vi "Single Char Seperator.vi"(8 "error in (no error)":errorcluster, 10 "String":string, 11 "VISA resource name":refnum<visa-resource-name>) -> (0 "error out":errorcluster, 3 "VISA resource name 2":refnum<visa-resource-name>)   [LabVIEW 2013]
panel:
  out "return count":u32
  # "This progarm seperates out strings of commands into single\ncharacters and writes them to the buffer one at a time.  Last I\nchecked, this worked fine.  It is possible that this may not be \nneeded in the future."
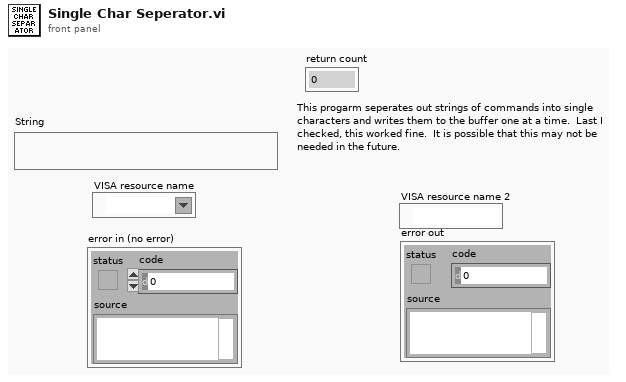
[diagram p1: front panel]
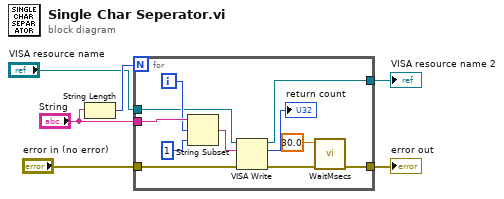
[diagram p0: block diagram]
diagram:
  n1 = String Length(string="String") -> (length=w6:i32)
  n2 = for {
    N: w6 -> [_]
    tunnel: "String" -> [w17]
    tunnel: "VISA resource name" -> [w14]
    tunnel: "error in (no error)" -> [w13]
    tunnel: [w12] -> w2
    tunnel: [w8] -> w1
    i -> [w16]
    n3 = String Subset(string=w17, offset (0)=w16, length (rest)=1 ("length (rest)")) -> (substring=w11:string)
    n4 = VISA Write(VISA resource name=w14, write buffer=w11, error in (no error)=w13) -> (VISA resource name out=w12:refnum<visa-resource-name>, return count=→"return count":u32, error out=w9:errorcluster)
    n5 = call "WaitMsecs.vi"("error in (no error)"=w9, "Wait Msecs"=30.0) -> ("error out"=w8:errorcluster)  [unwired: 9 in]
  }
  "VISA resource name 2" <- w2
  "error out" <- w1
